vi "MySystemUI.vi"() -> ()   [LabVIEW 2014, in "My System.lvclass"]
doc: "UI that will be called when the node is selected."
uses:
  My System.lvclass
  <vilib>/NI/Configuration Framework/Node/NodeRef.ctl
  <vilib>/NI/Configuration Framework/Node/NISE_CEF_Node.lvclass
  <vilib>/NI/AMC/Message Queue.ctl
  <vilib>/NI/AMC/Message.ctl
  <vilib>/NI/Tools/Keyed Array/KeyedArray.ctl
  <vilib>/NI/Configuration Framework/Node/UserEventRef.ctl
  <vilib>/NI/Configuration Framework/Controls/EventCluster.ctl
  <vilib>/NI/Tools/Keyed Array/Tools_KeyedArray.lvlib
  <vilib>/NI/AMC/AMC.lvlib
  <vilib>/NI/Configuration Framework/NISE_CEF_TreeControl.lvlib
panel:
  in  "user event":T1
  in  "main queue":T2
  in  "node ref":T3
types:
  T1 = typedef "NISE_CEF_Node.lvclass/UserEventRef.ctl" = refnum<user-event>
  T2 = typedef "AMC.lvlib/Message Queue.ctl" = refnum<queue>
  T3 = typedef "NISE_CEF_Node.lvclass/NodeRef.ctl" = refnum<data-value>
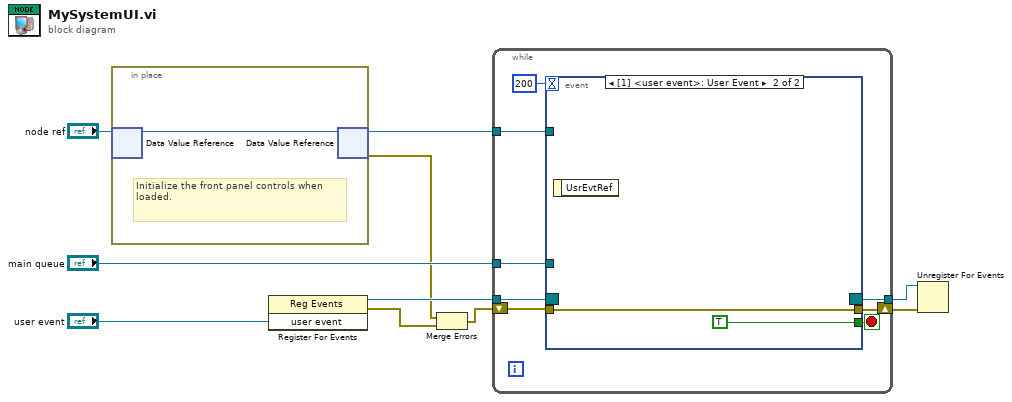
[diagram p0: block diagram]
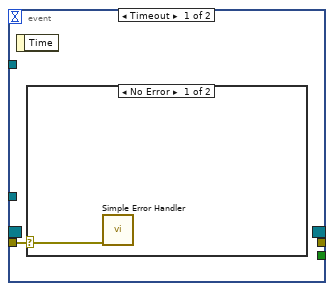
[diagram p2: hidden frame]
diagram:
  n1 = in-place {
    # "Initialize the front panel controls when loaded."
    n2 = in-place-dvr #1("node ref") -> (w11:refnum<class "NISE_CEF_Node.lvclass">)  [unwired: 1 out]
    n3 = in-place-dvr #1(w11) -> (w9:T3, w3:errorcluster)
  }
  n4 = register-events("user event") -> (reference out=w6:refnum<event-registration>, error out=w2:errorcluster)  [unwired: 2 in]
  n5 = Merge Errors(w3, w2) -> (w1:errorcluster)
  n6 = while {
    tunnel: w9 -> [w19]
    tunnel: "main queue" -> [w18]
    tunnel: w6 -> [w16]
    tunnel: [w15] -> w5
    shift-right: [w13] -> w4
    shift-left: w1 -> [w12]
    stop <- w14 stop-if-true
    n7 = event shown="[1] <user event>: User Event" {
      selector: w16 -> [_ _]
      dyn-events: [_ _] -> w15
      timeout: 200 -> [_ _]
      tunnel: w19 -> [_ _]
      tunnel: w18 -> [_ _]
      tunnel: [_ TRUE] -> w14
      tunnel: [_ w22] -> w13
      tunnel: w12 -> [w20 w22]
      event Timeout {
        n8 = event-data() -> ()  [unwired: 1 in, 1 out]
        n9 = case shown="No Error" w20 {
          selector: w20 -> [w21 _]
          frame No Error {
            n10 = call <vilib>:"Simple Error Handler.vi"("error in (no error)"=w21) -> ()  [unwired: 4 in, 5 out]
          }
          frame Error {
          }
        }
      }
      event User Event {
        n11 = event-data() -> ()  [unwired: 1 in, 1 out]
      }
    }
  }
  n12 = Unregister For Events(event registration refnum=w5, error in=w4) -> ()  [unwired: 1 out]
